vi "Drive_Cheezy.vi"(5 "Joystick. RB":bool, 8 "Joystick.Y_Axis_Left":dbl, 10 "Joystick.X_Axis_Right":dbl) -> (1 "Right_Motor_Out":dbl, 3 "Left_Motor_Out":dbl)   [LabVIEW 2018]
panel:
  in  "Joystick_In":T1
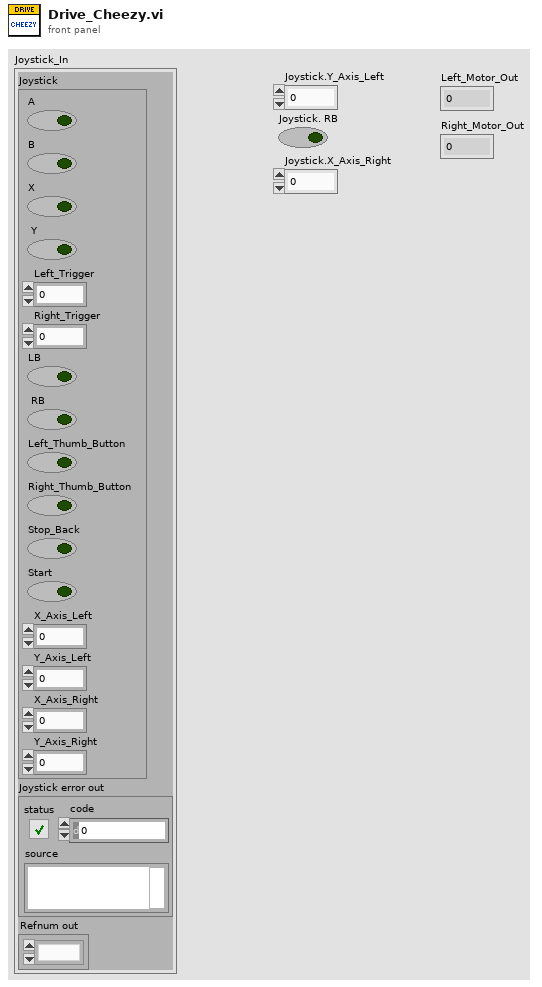
[diagram p1: front panel]
types:
  T1 = cluster{"Joystick":cluster{"A":bool, "B":bool, "X":bool, " Y":bool, "Left_Trigger":dbl, "Right_Trigger ":dbl, "LB":bool, " RB":bool, "Left_Thumb_Button":bool, "Right_Thumb_Button":bool, "Stop_Back":bool, "Start":bool, "X_Axis_Left":dbl, "Y_Axis_Left":dbl, "X_Axis_Right":dbl, "Y_Axis_Right":dbl}, "Joystick error out":errorcluster, "Refnum out":refnum<k1>}
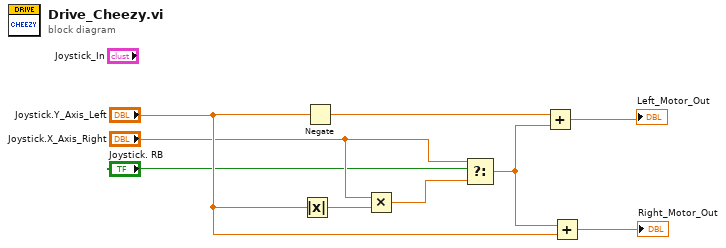
[diagram p0: block diagram]
diagram:
  n1 = Absolute Value(x="Joystick.Y_Axis_Left") -> (abs(x)=w5:dbl)
  n2 = Negate(x="Joystick.Y_Axis_Left") -> (-x=w9:dbl)
  n3 = Multiply(x="Joystick.X_Axis_Right", y=w5) -> (x*y=w4:dbl)
  n4 = Select(t="Joystick.X_Axis_Right", s="Joystick. RB", f=w4) -> (s? t:f=w7:dbl)
  n5 = Add(x=w9, y=w7) -> (x+y=→"Left_Motor_Out":dbl)
  n6 = Add(x=w7, y="Joystick.Y_Axis_Left") -> (x+y=→"Right_Motor_Out":dbl)
